vi "Update Filters Menu.vi"(8 "error in":errorcluster, 9 "ConfigInfo in":T1={"Data Tree Ref"=refnum, "FP Ref"=refnum, "Column Data Type"=[], "Search Clones Up To"=100, "SortOptions"={"Col.pri"=0, "RevDir.pri"=FALSE, "Col.sec"=0, "RevDir.sec"=FALSE}, "Group/Flat (0:group)"=FALSE, "CollapsedNodes"=[], "Show/Hide Cols"=[], "Filtered Paths"=[], "View"=enum."Group By Library", "File Extension Filters"=[], "Filter Global VIs"=FALSE, "Shared"=refnum, "Active Filters"=refnum, "Refresh Rate (ms)"=2000, "App Instance Ring Ref"=refnum, "Processing Q"=refnum, "VI Ref"=refnum}, 11 "Menu in":refnum<k9>) -> (0 "error out":errorcluster, 3 "Menu out":refnum<k9>)   [LabVIEW 2013, in "LVTM.lvlib"]
uses:
  LVTM.lvlib
  Controls_LVTM/LVTM_Config_Info.ctl
  Controls_LVTM/View.ctl
  Controls_LVTM/SharedDataDVR.ctl
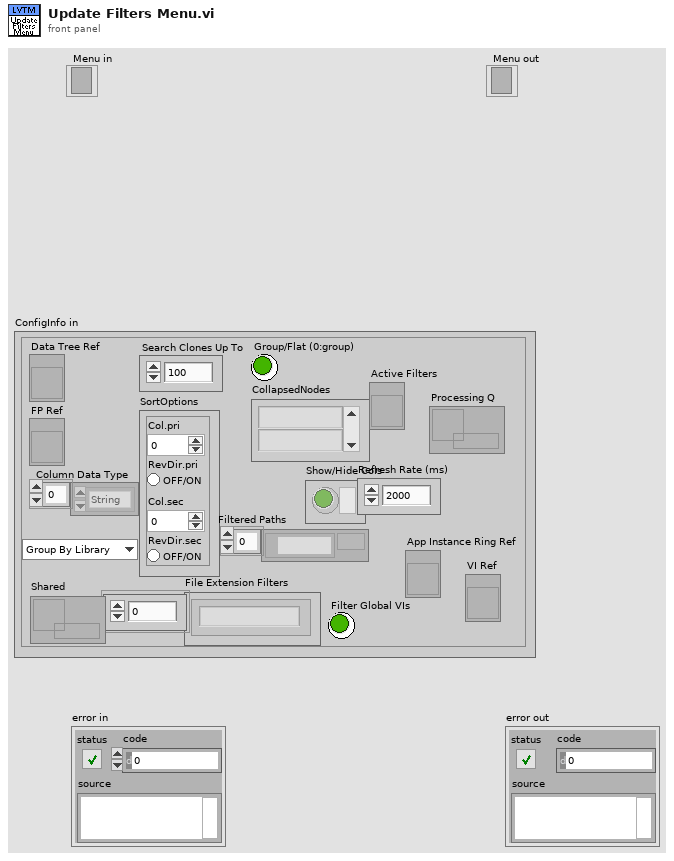
[diagram p1: front panel]
types:
  T1 = typedef "LVTM.lvlib/LVTM_Config_Info.ctl" = cluster{"Data Tree Ref":refnum<vi>, "FP Ref":refnum<vi>, "Column Data Type":enum16{"String", "Numeric"}[], "Search Clones Up To":i32, "SortOptions":cluster{"Col.pri":i32, "RevDir.pri":bool, "Col.sec":i32, "RevDir.sec":bool}, "Group/Flat (0:group)":bool, "CollapsedNodes":string[], "Show/Hide Cols":bool[], "Filtered Paths":path[], "View":T2, "File Extension Filters":string[], "Filter Global VIs":bool, "Shared":refnum<data-value>, "Active Filters":refnum<vi>, "Refresh Rate (ms)":i32, "App Instance Ring Ref":refnum<vi>, "Processing Q":refnum<queue>, "VI Ref":refnum<vi>}
  T2 = typedef "LVTM.lvlib/View.ctl" = enum16{"Group By Library", "Group By Folder", "Flat List"}
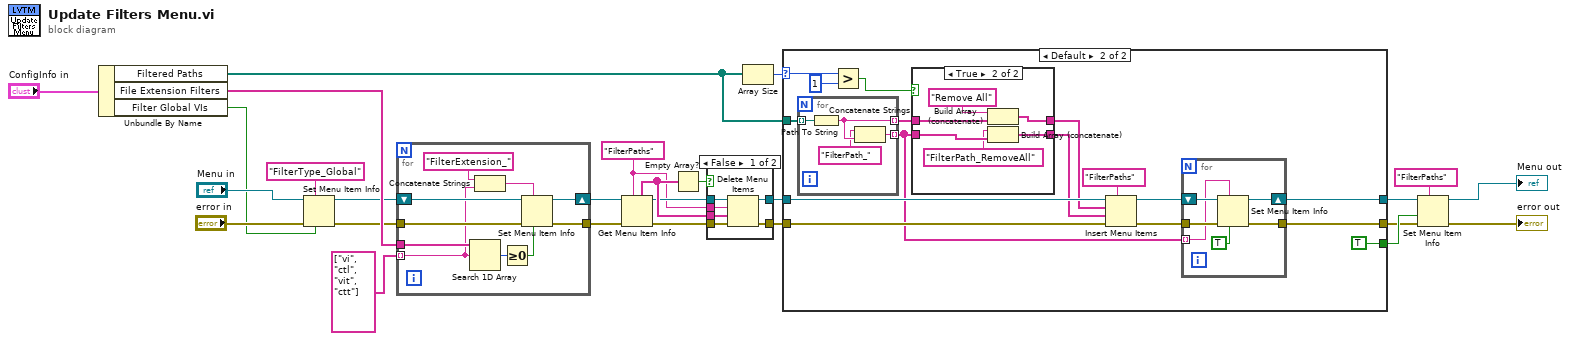
[diagram p0: block diagram]
diagram:
  w15 = "FilterPaths" ("menu tag")
  n1 = Unbundle By Name("ConfigInfo in") -> ("Filtered Paths"=w9:path[], "File Extension Filters"=w3:string[], "Filter Global VIs"=w4:bool)
  n2 = Set Menu Item Info(6:w4, 7:"FilterType_Global" ("item tag"), 8:"error in", 11:"Menu in") -> (0:w1:errorcluster, 3:w2:refnum<k9>)  [unwired: 3 in]
  n3 = for {
    tunnel: string[] ["vi", "ctl", "vit", "ctt"] -> [w29] mode=indexing
    tunnel: w1 -> [w35]
    tunnel: [w34] -> w17
    shift-right: [w33] -> w18
    shift-left: w2 -> [w36]
    tunnel: w3 -> [w30]
    n4 = Search 1D Array(1D array=w30, element=w29) -> (index of element=w28:i32)  [unwired: 1 in]
    n5 = Concatenate Strings("FilterExtension_" ("item tag"), w29) -> (w31:string)
    n6 = Greater Or Equal To 0?(x=w28) -> (x >= 0?=w27:bool)
    n7 = Set Menu Item Info(6:w27, 7:w31, 8:w35, 11:w36) -> (0:w34:errorcluster, 3:w33:refnum<k9>)  [unwired: 3 in]
  }
  n8 = Get Menu Item Info(7:w15, 8:w17, 11:w18) -> (0:w16:errorcluster, 3:w19:refnum<k9>, 5:w21:string[])  [unwired: 4 out]
  n9 = Empty Array?(array=w21) -> (empty?=w20:bool)
  n10 = case shown="False" w20 {
    tunnel: [w42 w44] -> w13
    tunnel: [w41 w43] -> w14
    tunnel: w21 -> [w40 _]
    tunnel: w15 -> [w39 _]
    tunnel: w16 -> [w38 w43]
    tunnel: w19 -> [w37 w44]
    frame False {
      n11 = Delete Menu Items(6:w38, 7:w40, 8:w39, 9:w37) -> (0:w41:errorcluster, 3:w42:refnum<k9>)
    }
    frame True {
    }
  }
  n12 = Array Size(array=w9) -> (size(s)=w12:i32)
  n13 = case shown="Default" w12 {
    selector: w12 -> [_ w58]
    tunnel: w13 -> [w45 w62]
    tunnel: [w46 w51] -> w24
    tunnel: w14 -> [w46 w61]
    tunnel: w9 -> [_ w60]
    tunnel: [w45 w50] -> w23
    tunnel: [_ TRUE ("enabled")] -> w26
    frame 0 {
    }
    frame Default {
      n14 = for {
        tunnel: w60 -> [w80] mode=indexing
        tunnel: [w79] -> w54 mode=indexing
        tunnel: [w78] -> w47 mode=indexing
        n15 = Path To String(path=w80) -> (string=w79:string)
        n16 = Concatenate Strings("FilterPath_" ("menu tag"), w79) -> (w78:string)
      }
      n17 = Greater?(x=w58, y=1) -> (0:w56:bool)
      n18 = case shown="True" w56 {
        tunnel: [w70 w73] -> w55
        tunnel: w54 -> [w70 w76]
        tunnel: [w69 w74] -> w53
        tunnel: w47 -> [w69 w75]
        frame False {
        }
        frame True {
          n19 = Build Array (concatenate)("Remove All" ("menu tag"), w76) -> (w73:string[])
          n20 = Build Array (concatenate)("FilterPath_RemoveAll" ("menu tag"), w75) -> (w74:string[])
        }
      }
      n21 = Insert Menu Items(5:"FilterPaths" ("menu tag"), 6:w61, 7:w53, 8:w55, 9:w62) -> (0:w49:errorcluster, 3:w48:refnum<k9>)  [unwired: 1 in, 1 out]
      n22 = for {
        tunnel: w49 -> [w67]
        tunnel: [w66] -> w51
        shift-right: [w65] -> w50
        shift-left: w48 -> [w68]
        tunnel: w47 -> [w63] mode=indexing
        n23 = Set Menu Item Info(6:TRUE ("checked"), 7:w63, 8:w67, 11:w68) -> (0:w66:errorcluster, 3:w65:refnum<k9>)  [unwired: 3 in]
      }
    }
  }
  n24 = Set Menu Item Info(7:"FilterPaths" ("menu tag"), 8:w24, 9:w26, 11:w23) -> (0:→"error out":errorcluster, 3:→"Menu out":refnum<k9>)  [unwired: 3 in]
